vi "Heat Main.vi"(0 "GEA2 Reference In":refnum<k24>, 5 "Inlet Temperature":dbl, 9 "Outlet Temperature":dbl, 11 "Error In":errorcluster) -> (4 "Heat Control out":T1, 15 "Error Out":errorcluster)   [LabVIEW 2016]
uses:
  Q:/Common/DLLs/GEA3/GeaCommunication.dll
  Common/DLLs/GEA3/GeaCommunication.dll
  Controls/Auto_Heat Control_Out.ctl
  Common/LabVIEW GEA2 Toolkit/LabVIEW_GEA2_Toolkit.lvlibp/type defs/Source_Destination.ctl
  Common/LabVIEW GEA2 Toolkit/LabVIEW_GEA2_Toolkit.lvlibp
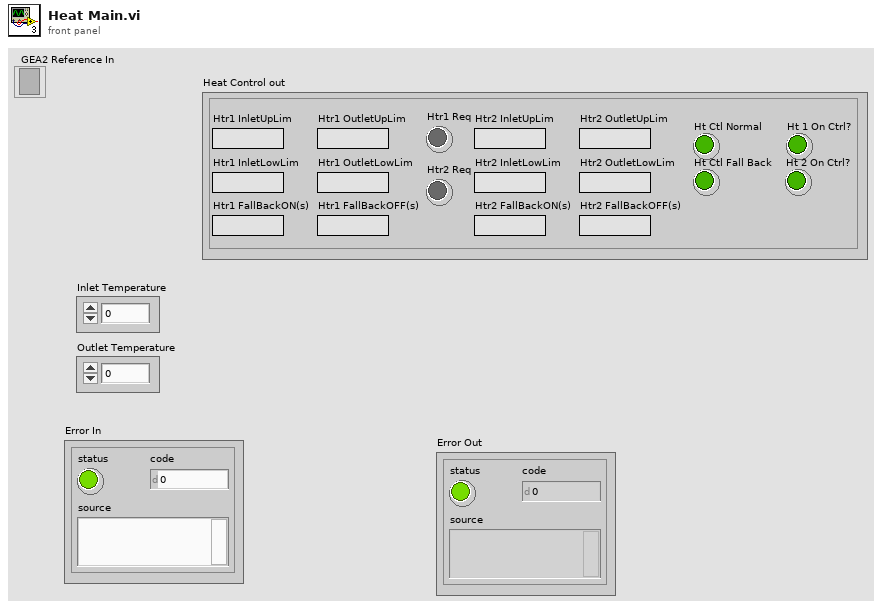
[diagram p1: front panel]
types:
  T1 = typedef "Auto_Heat Control_Out.ctl" = cluster{"Htr1 InletLowLim":string, "Htr1 InletUpLim":string, "Htr1 OutletLowLim":string, "Htr1 OutletUpLim":string, "Htr1 FallBackON(s)":string, "Htr1 FallBackOFF(s)":string, "Htr1 Req":bool, "Htr2 InletLowLim":string, "Htr2 InletUpLim":string, "Htr2 OutletLowLim":string, "Htr2 OutletUpLim":string, "Htr2 FallBackON(s)":string, "Htr2 FallBackOFF(s)":string, "Htr2 Req":bool, "Ht Ctl Normal":bool, "Ht Ctl Fall Back":bool, "Ht 1 On Ctrl?":bool, "Ht 2 On Ctrl?":bool}
  T2 = typedef "LabVIEW_GEA2_Toolkit.lvlibp/Source_Destination.ctl" = cluster{"Source":u8, "Destination":u8}
  T3 = typedef "LabVIEW_GEA2_Toolkit.lvlibp/ERD Read Data Out.ctl" = cluster{"ERD Number":u16, "Data":string}
  T4 = typedef "Heat Control.ctl" = cluster{"Htr1 InletLowLim":string, "Htr1 InletUpLim":string, "Htr1 OutletLowLim":string, "Htr1 OutletUpLim":string, "Htr1 FallBackON(s)":string, "Htr1 FallBackOFF(s)":string, "Htr1":bool, "Htr2 InletLowLim":string, "Htr2 InletUpLim":string, "Htr2 OutletLowLim":string, "Htr2 OutletUpLim":string, "Htr2 FallBackON(s)":string, "Htr2 FallBackOFF(s)":string, "Htr2":bool}
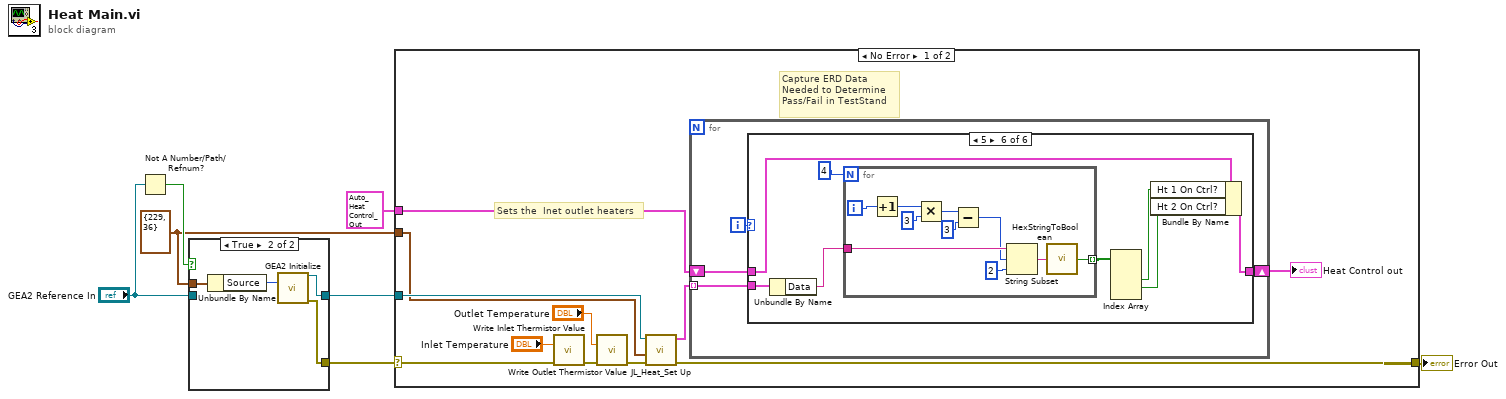
[diagram p0: block diagram]
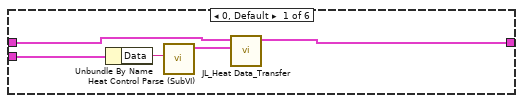
[diagram p2: hidden frame]
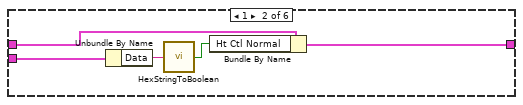
[diagram p3: hidden frame]
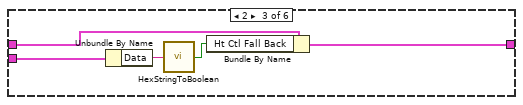
[diagram p4: hidden frame]
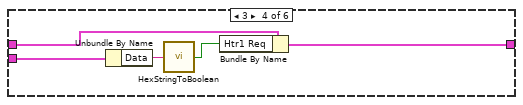
[diagram p5: hidden frame]
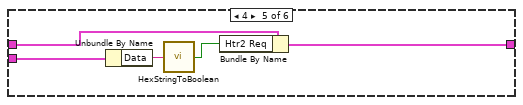
[diagram p6: hidden frame]
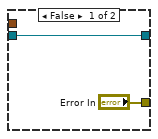
[diagram p8: hidden frame]
diagram:
  w4 = T2 {"Source"=229, "Destination"=36} ("GEA Inputs")
  n1 = Not A Number/Path/Refnum?(number/path/refnum="GEA2 Reference In") -> (NaN/Path/Refnum?=w7:bool)
  n2 = case shown="True" w7 {
    tunnel: w4 -> [_ w13]
    tunnel: [w9 w11] -> w3
    tunnel: "GEA2 Reference In" -> [w9 _]
    tunnel: ["Error In" w10] -> w5
    frame False {
    }
    frame True {
      n3 = Unbundle By Name(w13) -> ("Source"=w12:u8)
      n4 = call "GEA2 Initialize.vi"("Source Address"=w12) -> ("GEA2 Reference Out"=w11:refnum<k24>, "error out"=w10:errorcluster)  [unwired: 12 in, 1 out]
    }
  }
  n5 = case shown="No Error" w5 {
    selector: w5 -> [w15 w72]
    tunnel: w4 -> [w23 _]
    tunnel: [w22 w72] -> w2
    tunnel: w3 -> [w24 _]
    tunnel: T1 {"Htr1 InletLowLim"="190", "Htr1 InletUpLim"="238", "Htr1 OutletLowLim"="120", "Htr1 OutletUpLim"="128", "Htr1 FallBackON(s)"="70", "Htr1 FallBackOFF(s)"="40", "Htr1 Req"=TRUE, "Htr2 InletLowLim"="195", "Htr2 InletUpLim"="268", "Htr2 OutletLowLim"="120", "Htr2 OutletUpLim"="128", "Htr2 FallBackON(s)"="71", "Htr2 FallBackOFF(s)"="41", "Htr2 Req"=TRUE, "Ht Ctl Normal"=FALSE, "Ht Ctl Fall Back"=FALSE, "Ht 1 On Ctrl?"=FALSE, "Ht 2 On Ctrl?"=FALSE} ("Heat Control out") -> [w21 _]
    frame No Error {
      # "Capture ERD Data \nNeeded to Determine \nPass/Fail in TestStand"
      # "Sets the  Inet outlet heaters"
      n6 = call "Write Inlet Thermistor Value.vi"("Inlet Temperature"="Inlet Temperature", "Error In"=w15) -> ("Error Out"=w18:errorcluster)  [unwired: 13 in]
      n7 = call "Write Outlet Thermistor Value.vi"("Outlet Temperature"="Outlet Temperature", "Error In"=w18) -> ("Error Out"=w14:errorcluster)  [unwired: 13 in]
      n8 = call "JL_Heat_Set Up.vi"("error in (no error)"=w14, "GEA Inputs"=w23, ".NET Refnum in"=w24) -> ("error out"=w22:errorcluster, "ERD Data Out"=w20:T3[])  [unwired: 7 in]
      n9 = for {
        tunnel: w20 -> [w26] mode=indexing
        shift-right: [w28] -> w19
        shift-left: w21 -> [w27]
        i -> [w25]
        n10 = case shown="5" w25 {
          tunnel: [w29 w34 w39 w44 w49 w55] -> w28
          tunnel: w27 -> [w31 w36 w40 w45 w50 w54]
          tunnel: w26 -> [w33 w38 w43 w48 w53 w59]
          frame 0, Default {
            n11 = Unbundle By Name(w33) -> ("Data"=w32:string)
            n12 = call "Heat Control Parse (SubVI).vi"("Data"=w32) -> ("Heat Control out"=w30:T4)  [unwired: 10 in]
            n13 = call "JL_Heat Data_Transfer.vi"("Heat Control in"=w30, "Heat Control out 3"=w31) -> ("Heat Control out"=w29:T1)  [unwired: 9 in]
          }
          frame 1 {
            n14 = Unbundle By Name(w38) -> ("Data"=w37:string)
            n15 = call "HexStringToBoolean.vi"("Hex String"=w37) -> ("Boolean"=w35:bool)
            n16 = Bundle By Name(cluster=w36, "Ht Ctl Normal"=w35) -> (w34:T1)
          }
          frame 2 {
            n17 = Unbundle By Name(w43) -> ("Data"=w42:string)
            n18 = call "HexStringToBoolean.vi"("Hex String"=w42) -> ("Boolean"=w41:bool)
            n19 = Bundle By Name(cluster=w40, "Ht Ctl Fall Back"=w41) -> (w39:T1)
          }
          frame 3 {
            n20 = Unbundle By Name(w48) -> ("Data"=w47:string)
            n21 = call "HexStringToBoolean.vi"("Hex String"=w47) -> ("Boolean"=w46:bool)
            n22 = Bundle By Name(cluster=w45, "Htr1 Req"=w46) -> (w44:T1)
          }
          frame 4 {
            n23 = Unbundle By Name(w53) -> ("Data"=w52:string)
            n24 = call "HexStringToBoolean.vi"("Hex String"=w52) -> ("Boolean"=w51:bool)
            n25 = Bundle By Name(cluster=w50, "Htr2 Req"=w51) -> (w49:T1)
          }
          frame 5 {
            n26 = Unbundle By Name(w59) -> ("Data"=w58:string)
            n27 = for {
              N: 4 -> [_]
              tunnel: w58 -> [w71]
              tunnel: [w68] -> w61 mode=indexing
              i -> [w63]
              n28 = Increment(x=w63) -> (x+1=w62:i32)
              n29 = Multiply(x=w62, y=3) -> (x*y=w66:i32)
              n30 = Subtract(x=w66, y=3) -> (x-y=w64:i32)
              n31 = String Subset(string=w71, offset (0)=w64, length (rest)=2 ("length (rest)")) -> (substring=w69:string)
              n32 = call "HexStringToBoolean.vi"("Hex String"=w69) -> ("Boolean"=w68:bool)
            }
            n33 = Index Array(array=w61) -> (element #2=w57:bool, element #3=w56:bool)  [unwired: 4 in, 2 out]
            n34 = Bundle By Name(cluster=w54, "Ht 1 On Ctrl?"=w57, "Ht 2 On Ctrl?"=w56) -> (w55:T1)
          }
        }
      }
      "Heat Control out" <- w19
    }
    frame Error {
    }
  }
  "Error Out" <- w2
